vi "create available tags menu.vi"(8 "error in":errorcluster, 9 "channel to map to":refnum<class "TBM channel.lvclass">, 10 "MenuRef":refnum<k9>, 11 "engine configuration in":refnum<class "engine configuration.lvclass">) -> (0 "error out":errorcluster, 3 "engine configuration out":refnum<class "engine configuration.lvclass">)   [LabVIEW 2013, in "control module editor.lvclass"]
uses:
  control module editor.lvclass
  <vilib>/NI/Module Execution Interface/Engine Configuration/engine configuration.lvclass
  <vilib>/NI/Tag Bus Module Framework/channel/TBM channel.lvclass
  <vilib>/NI/Tag Bus/tag/tag descriptor.lvclass/tag descriptor.ctl
  <vilib>/NI/Tag Bus/tag/read tag name.vi
  <vilib>/NI/Tag Bus/tag/tag descriptor.lvclass
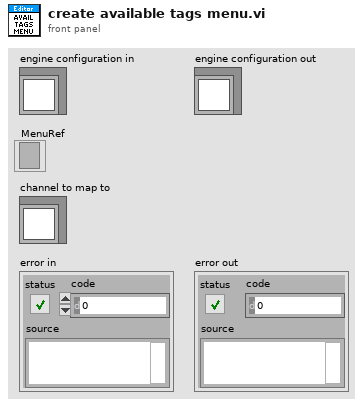
[diagram p1: front panel]
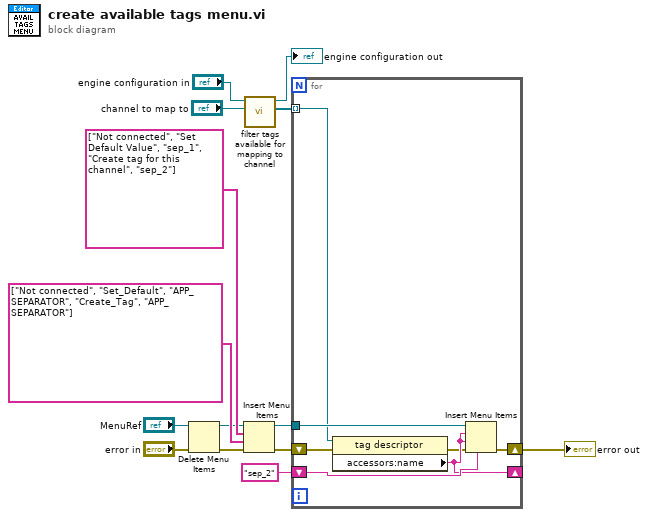
[diagram p0: block diagram]
diagram:
  n1 = Delete Menu Items(6:"error in", 9:"MenuRef") -> (0:w2:errorcluster, 3:w3:refnum<k9>)  [unwired: 2 in]
  n2 = Insert Menu Items(6:w2, 7:string[] ["Not connected", "Set_Default", "APP_SEPARATOR", "Create_Tag", "APP_SEPARATOR"] ("item tags"), 8:string[] ["Not connected", "Set Default Value", "sep_1", "Create tag for this channel", "sep_2"] ("item names"), 9:w3) -> (0:w7:errorcluster, 3:w10:refnum<k9>)  [unwired: 2 in, 1 out]
  n3 = call <vilib>:"filter tags available for mapping to channel.vi"("channel to map to"="channel to map to", "engine configuration in"="engine configuration in") -> ("filtered tags"=w9:refnum<class "tag descriptor.lvclass">[], "engine configuration out"=→"engine configuration out":refnum<class "engine configuration.lvclass">)  [unwired: 8 in]
  n4 = for {
    tunnel: w10 -> [w21]
    tunnel: w9 -> [w20] mode=indexing
    shift-right: [w18] -> _
    shift-left: "sep_2" -> [w19]
    shift-right: [w15] -> w6
    shift-left: w7 -> [w17]
    n5 = property class="tag descriptor"(reference=w20, error in=w17) -> (error out=w16:errorcluster, "accessors:name"=w18:string)  [unwired: 1 out]
    n6 = Insert Menu Items(4:w19, 6:w16, 7:w18, 8:w18, 9:w21) -> (0:w15:errorcluster)  [unwired: 1 in, 2 out]
  }
  "error out" <- w6
